vi "meta PID - Wave - V1.vi"(4 "default output":dbl=300.0, 6 "input parameter":dbl=300.0, 7 "control?":bool, 8 "lower limit":dbl=-inf, 9 "upper limit":dbl=inf, 10 "sweep folder path":path, 11 "ctl name dispatch":T1) -> (0 "output":dbl, 1 "frequencies":dbl[](array[numeric]), 2 "temperatures":dbl[](array[numeric]), 3 "ok":bool)   [LabVIEW 2015]
uses:
  ctl -- name dispatcher -- action.ctl
  next chunk read-write PID -- action.ctl
  file -- 9w path.vi
  array -- find index - real.vi
  array -- interpolate -- i.vi
  Q - not nan -- real.vi
  <vilib>/Utility/libraryn.llb/Check if File or Folder Exists.vi
  file -- read list of lines.vi
  parse -- find first line.vi
  parse -- get list of matches -- numbers.vi
  <vilib>/Utility/file.llb/Write To Spreadsheet File.vi
  <vilib>/Utility/file.llb/Write To Spreadsheet File (string).vi
  <vilib>/gmath/function.llb/Binomial Coefficient.vi
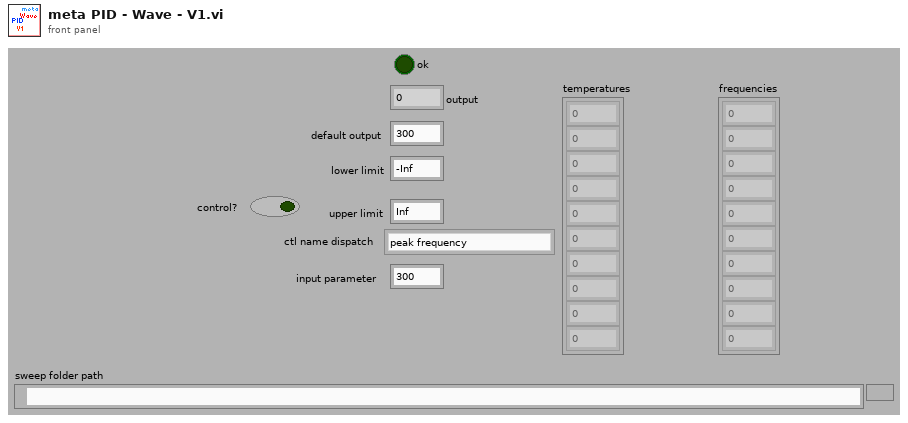
[diagram p1: front panel]
types:
  T1 = typedef "ctl -- name dispatcher -- action.ctl" = enum16{"peak frequency", "peak frequency DUMP", "peak gamma DUMP", "peak gamma", "peak frequency TEST", "peak gamma TEST", "ultrasonic power", "time in gamma", "set temperature ", "set temperature timer", "peak default gamma", "last scan file", "peak freq gamma TEST", "peak NAMES", "errors", "P_I_D", "P", "I", "D", "power vs time", "power vs time TIMER", "void", "power log", "set temperature - SINE", "itc ltc log", "peak - time in gamma"}
  T2 = typedef "next chunk read-write PID -- action.ctl" = enum16{"read", "interpolate", "append col", "write", "write PID col", "append PID col", "interpolate - bezier"}
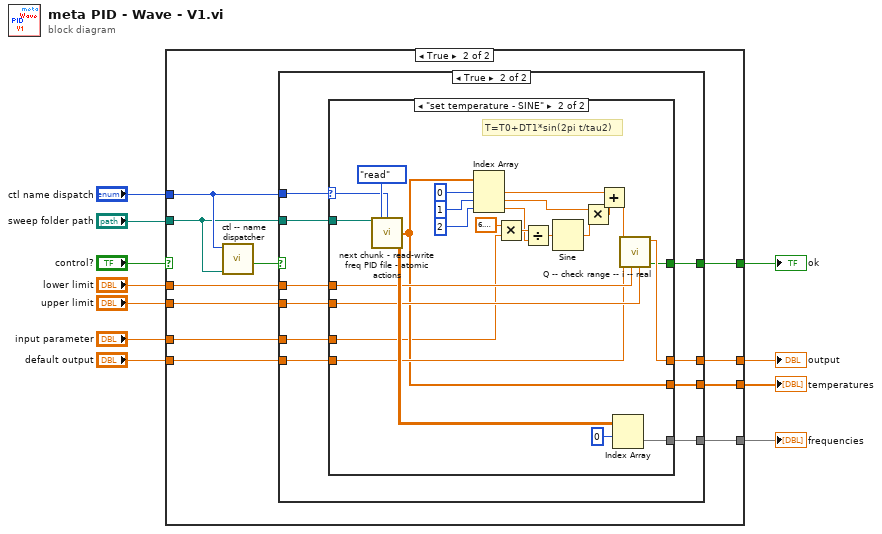
[diagram p0: block diagram]
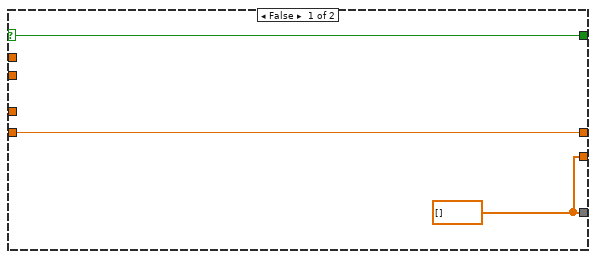
[diagram p2: hidden frame]
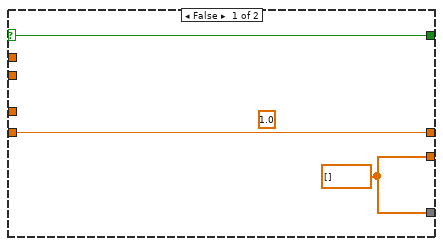
[diagram p3: hidden frame]
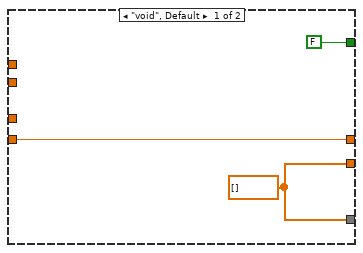
[diagram p4: hidden frame]
diagram:
  n1 = case shown="True" "control?" {
    selector: "control?" -> [w13 _]
    tunnel: "sweep folder path" -> [_ w16]
    tunnel: "input parameter" -> [_ w25]
    tunnel: [w12 w24] -> w8
    tunnel: [w14 w23] -> w7
    tunnel: [w14 w22] -> w6
    tunnel: "lower limit" -> [_ w21]
    tunnel: "upper limit" -> [_ w20]
    tunnel: [w13 w19] -> w3
    tunnel: "ctl name dispatch" -> [_ w17]
    tunnel: "default output" -> [w12 w15]
    frame False {
      w14 = dbl[] [] ("temperatures")
    }
    frame True {
      n2 = call "ctl -- name dispatcher.vi"("sweep folder path"=w16, "ctl name dispatch"=w17) -> ("file or folder exists?"=w18:bool)  [unwired: 7 in, 2 out]
      n3 = case shown="True" w18 {
        selector: w18 -> [w27 _]
        tunnel: w16 -> [_ w38]
        tunnel: w17 -> [_ w29]
        tunnel: w25 -> [_ w30]
        tunnel: [w26 w37] -> w24
        tunnel: [w28 w31] -> w23
        tunnel: [w28 w36] -> w22
        tunnel: w21 -> [_ w35]
        tunnel: w20 -> [_ w34]
        tunnel: [w27 w33] -> w19
        tunnel: w15 -> [w26 w32]
        frame False {
          w28 = dbl[] [] ("temperatures")
          (unwired) 1.0 ("upper")
        }
        frame True {
          n4 = case shown="\"set temperature - SINE\"" w29 {
            selector: w29 -> [_ w45]
            tunnel: w38 -> [_ w65]
            tunnel: [w40 w64] -> w37
            tunnel: [w41 w62] -> w36
            tunnel: w35 -> [_ w60]
            tunnel: w34 -> [_ w59]
            tunnel: [FALSE w58] -> w33
            tunnel: w32 -> [w40 w57]
            tunnel: [w41 w56] -> w31
            tunnel: w30 -> [_ w51]
            frame "void", Default {
              w41 = dbl[] [] ("temperatures")
            }
            frame "set temperature - SINE" {
              # "T=T0+DT1*sin(2pi t/tau2)"
              n5 = call "next chunk - read-write freq PID file - atomic actions .vi"("sweep folder path"=w65, "PID action"=next_chunk_read-write_PID_--_action."read", "ctl kind IN"=w45) -> ("temperatures"=w56:dbl[], "frequencies"=w61:dbl[][])  [unwired: 8 in, 3 out]
              n6 = Index Array(array=w56, index #1=0 ("index"), index #2=1 ("index"), index #3=2 ("index")) -> (element #1=w55:dbl, element #2=w53:dbl, element #3=w49:dbl)
              n7 = Multiply(x=6.283185307179586, y=w51) -> (x*y=w50:dbl)
              n8 = Divide(x=w50, y=w49) -> (x/y=w48:dbl)
              n9 = Sine(x=w48) -> (sin(x)=w47:dbl)
              n10 = Multiply(x=w53, y=w47) -> (x*y=w54:dbl)
              n11 = Add(x=w55, y=w54) -> (x+y=w46:dbl)
              n12 = Index Array(array=w61, index (row)=0) -> (element=w62:dbl[])  [unwired: 1 in]
              n13 = call "Q -- check range -- i -- real.vi"("upper"=w59, "lower"=w60, "default"=w57, "number"=w46) -> ("in range?"=w58:bool, "number in range"=w64:dbl)  [unwired: 5 in, 1 out]
            }
          }
        }
      }
    }
  }
  "output" <- w8
  "temperatures" <- w7
  "frequencies" <- w6
  "ok" <- w3
